vi "CTRE_Phoenix_CANcoder_ConfigMagnetOffset.vi"(6 "timeoutMs":i32, 8 "error in":errorcluster, 10 "Magnet Offset (Degrees)":dbl, 11 "CTRE_CANcoder_DeviceRef":T1) -> (0 "error out":errorcluster, 3 "CTRE_CANcoder_DeviceRef":T1)   [LabVIEW 2020]
doc: "Adjusts the zero point for the absolute position register.\nThe absolute position of the sensor will always have a discontinuity (360 -> 0 deg) or (+180 -> -180) and a hard-limited mechanism may have such a discontinuity in its functional range.\nIn which case use this config to move the discontinuity outside of the function range.\n\n<b>Magnet Offset (Degrees)</b> Offset in degrees (unit string and coefficient DO NOT apply for this config).\n<b>timeoutMs</b> Timeout value in ms. If nonzero, function will wait for config success and report an error if it times out. If zero, no blocking or checking is performed."
uses:
  <vilib>/Rock Robotics/WPI/ThirdParty/Phoenix-LabVIEW/CANCoder/Controls/CTRE_Phoenix_CANcoder_DeviceRef.ctl
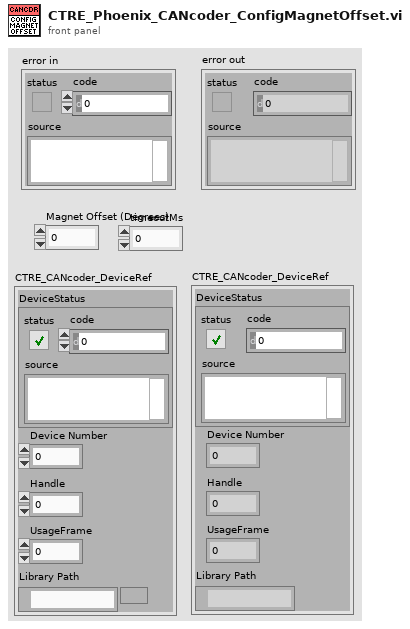
[diagram p1: front panel]
types:
  T1 = typedef "CTRE_Phoenix_CANcoder_DeviceRef.ctl" = cluster{"DeviceStatus":errorcluster, "Device Number":u8, "Handle":u64, "UsageFrame":u32, "Library Path":path}
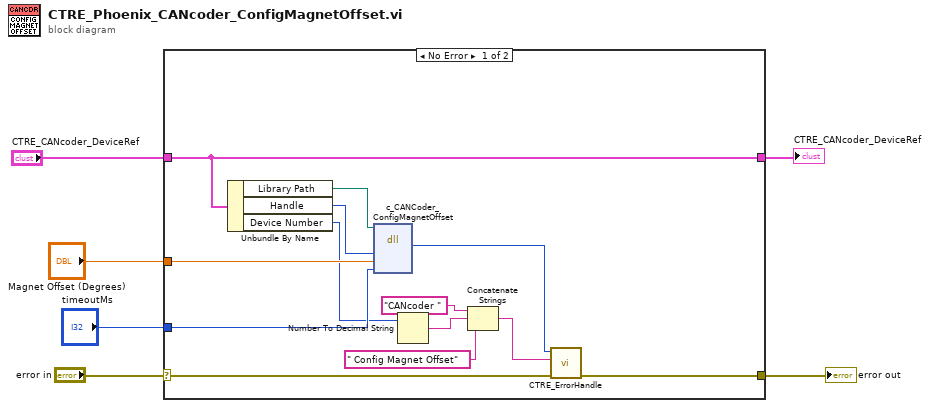
[diagram p0: block diagram]
diagram:
  n1 = case shown="No Error" "error in" {
    selector: "error in" -> [w16 w21]
    tunnel: "CTRE_CANcoder_DeviceRef" -> [w17 w20]
    tunnel: [w15 w21] -> w5
    tunnel: [w17 w20] -> w1
    tunnel: "timeoutMs" -> [w13 _]
    tunnel: "Magnet Offset (Degrees)" -> [w12 _]
    frame No Error {
      n2 = Unbundle By Name(w17) -> ("Library Path"=w19:path, "Handle"=w18:u64, "Device Number"=w7:u8)
      n3 = dll-call lib="?" fn="c_CANCoder_ConfigMagnetOffset"(path in=w19, "handle"=w18, "offsetDegrees"=w12, "timeoutMs"=w13) -> ("CTR_Code"=w14:i8)  [unwired: 5 in, 2 out]
      n4 = Number To Decimal String(number=w7) -> (decimal integer string=w11:string)  [unwired: 1 in]
      n5 = Concatenate Strings("CANcoder " ("string"), w11, " Config Magnet Offset" ("string")) -> (w8:string)
      n6 = call <vilib>:"CTRE_ErrorHandle.vi"("error in"=w16, "origin"=w8, "code"=w14) -> ("error out"=w15:errorcluster)  [unwired: 8 in]
    }
    frame Error {
    }
  }
  "error out" <- w5
  "CTRE_CANcoder_DeviceRef" <- w1
